vi "UDP_Packet_Inquiry.vi"(10 "Remote Port":u16=61557, 11 "UDP_Packet":T2 {"Command" format="%.0x"}) -> (2 "List":T1(array[cluster]) {"AmpUnit" format="%.0x"; "AnalogCH" format="%.0x"; "USB" format="%.0x"; "IP_Busy" format="%.0x"; "Count" format="%.0x"})   [LabVIEW 2017]
uses:
  UDP_Packet.ctl
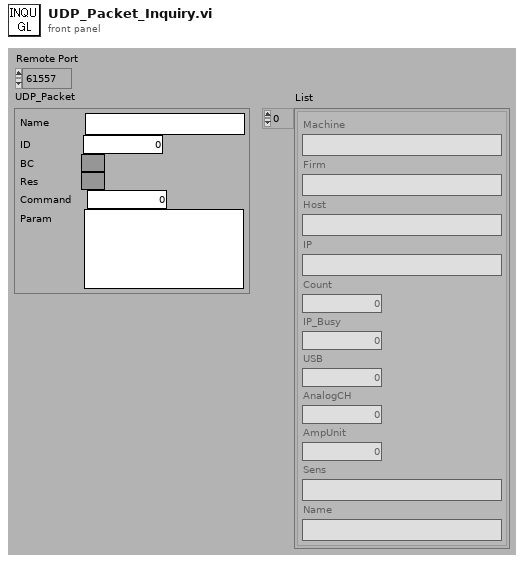
[diagram p1: front panel]
types:
  T1 = cluster{"Machine":string, "Firm":string, "Host":string, "IP":string, "Count":u32, "IP_Busy":u32, "USB":u32, "AnalogCH":u32, "AmpUnit":u32, "Sens":string, "Name":string}[]
  T2 = typedef "UDP_Packet.ctl" = cluster{"Name":string, "ID":u32, "BC":bool, "Res":bool, "Command":u32, "Param":string}
  T3 = enum16{"GL800", "GL200", "TH", "VT", "AC", "AT", "LU", "CO2", "TSR", "CO2_TH", "CO2_LU", "LU_TH"}[]
  T4 = cluster{"time":timestamp, "Inquiry":cluster{"Machine":string, "Firm":string, "Host":string, "IP":cluster{"A":u8, "B":u8, "C":u8, "D":u8}, "Count":u32, "IP_Busy":u32, "USB":u32, "AnalogCH":u32, "AmpUnit":u32, "Sens":cluster{"ID1":u16, "ID2":u16}, "Name":string}}
  T5 = cluster{"Machine":string, "Firm":string, "Host":string, "IP":cluster{"A":u8, "B":u8, "C":u8, "D":u8}, "Count":u32, "IP_Busy":u32, "USB":u32, "AnalogCH":u32, "AmpUnit":u32, "Sens":cluster{"ID1":u16, "ID2":u16}, "Name":string}
  T6 = cluster{timestamp, "Inquiry":cluster{"Machine":string, "Firm":string, "Host":string, "IP":cluster{"A":u8, "B":u8, "C":u8, "D":u8}, "Count":u32, "IP_Busy":u32, "USB":u32, "AnalogCH":u32, "AmpUnit":u32, "Sens":cluster{"ID1":u16, "ID2":u16}, "Name":string}}
  T7 = cluster{"time":timestamp, "Inquiry":cluster{"Machine":string, "Firm":string, "Host":string, "IP":cluster{"A":u8, "B":u8, "C":u8, "D":u8}, "Count":u32, "IP_Busy":u32, "USB":u32, "AnalogCH":u32, "AmpUnit":u32, "Sens":cluster{"ID1":u16, "ID2":u16}, "Name":string}}[]
  T8 = cluster{"Host":string, "IP":cluster{"A":u8, "B":u8, "C":u8, "D":u8}}
  T9 = cluster{"Machine":string, "Host":string, "IP":cluster{"A":u8, "B":u8, "C":u8, "D":u8}, "Inquiry":cluster{"Machine":string, "Firm":string, "Host":string, "IP":cluster{"A":u8, "B":u8, "C":u8, "D":u8}, "Count":u32, "IP_Busy":u32, "USB":u32, "AnalogCH":u32, "AmpUnit":u32, "Sens":cluster{"ID1":u16, "ID2":u16}, "Name":string}}
  T10 = cluster{"Machine":string, "Host":string, "IP":cluster{"A":u8, "B":u8, "C":u8, "D":u8}, "Inquiry":cluster{"Machine":string, "Firm":string, "Host":string, "IP":cluster{"A":u8, "B":u8, "C":u8, "D":u8}, "Count":u32, "IP_Busy":u32, "USB":u32, "AnalogCH":u32, "AmpUnit":u32, "Sens":cluster{"ID1":u16, "ID2":u16}, "Name":string}}[]
  T11 = cluster{"Machine":string, "Firm":string, "Host":string, string, "Count":u32, "IP_Busy":u32, "USB":u32, "AnalogCH":u32, "AmpUnit":u32, string, "Name":string}
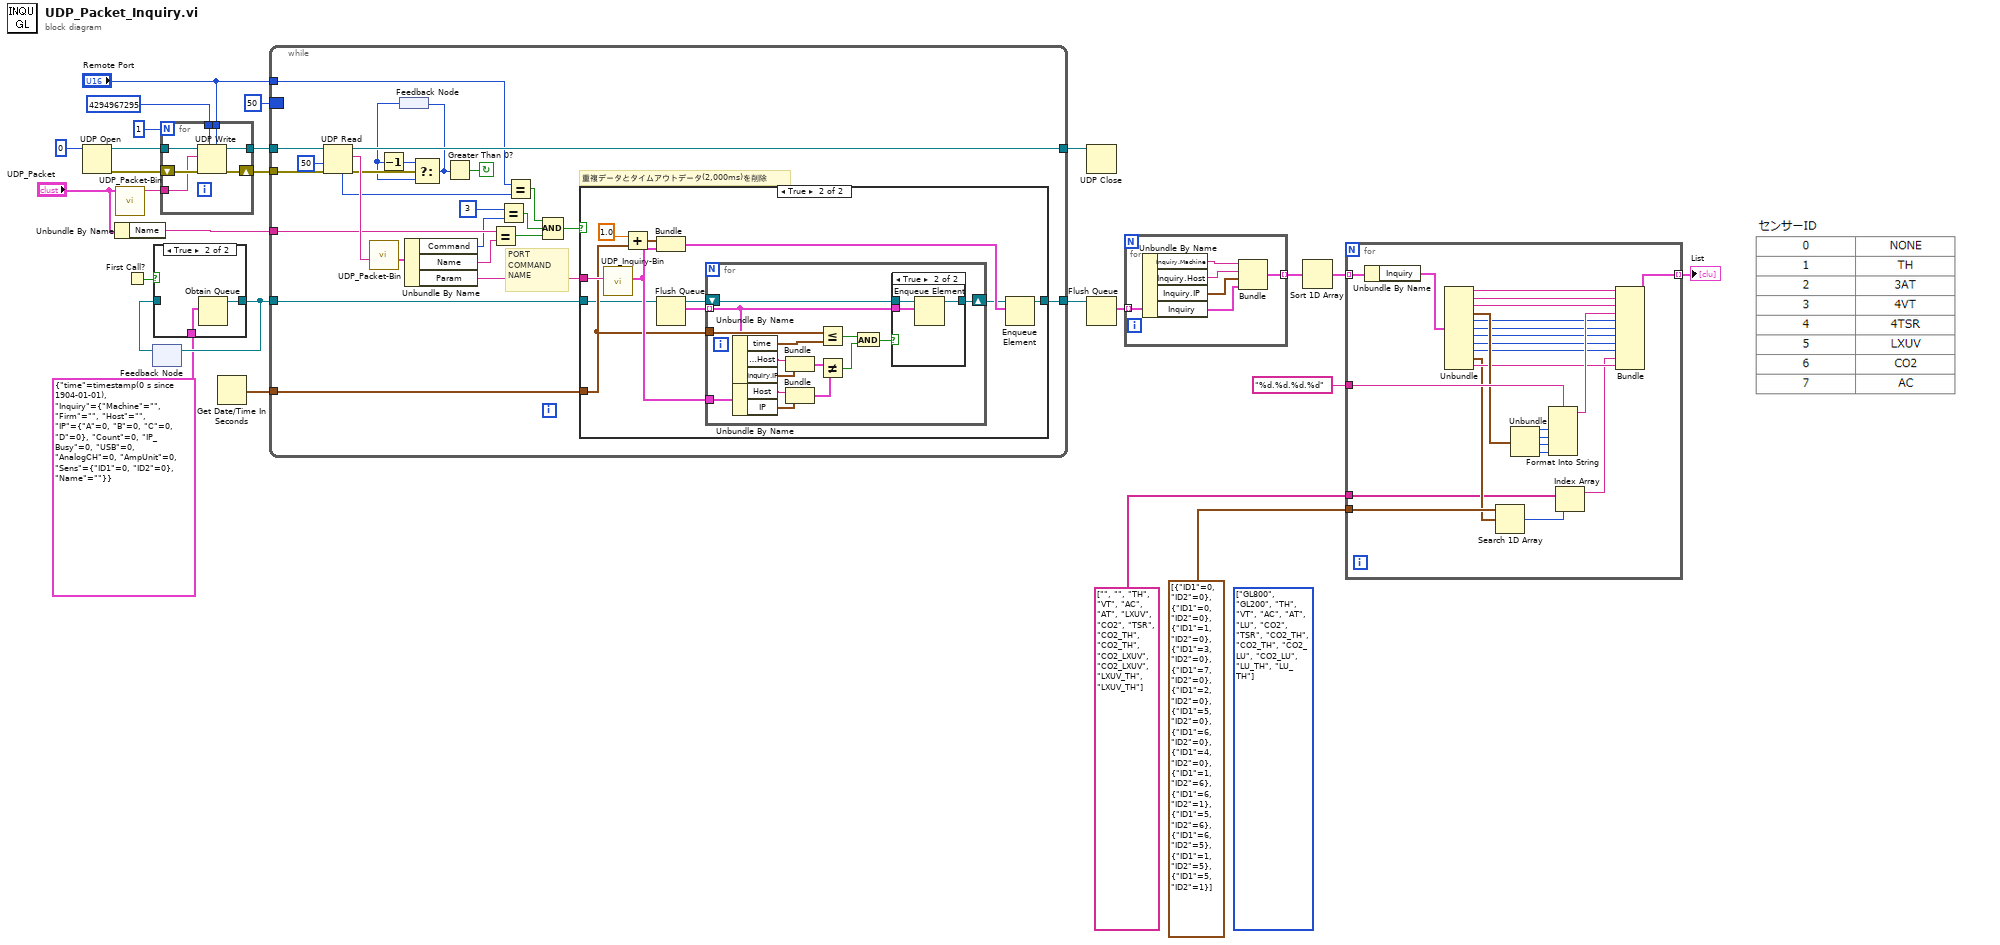
[diagram p0: block diagram]
diagram:
  (unwired) T3 [enum."GL800", enum."GL200", enum."TH", enum."VT", enum."AC", enum."AT", enum."LU", enum."CO2", enum."TSR", enum."CO2_TH", enum."CO2_TH", enum."CO2_LU", enum."CO2_LU", enum."LU_TH", enum."LU_TH"] items=["GL800", "GL200", "TH", "VT", "AC", "AT", "LU", "CO2", "TSR", "CO2_TH", "CO2_LU", "LU_TH"]
  n1 = UDP Open(11:u16 0 ("port")) -> (port=w26:refnum<k16>, 0:w25:errorcluster)  [unwired: 1 in, 4 out]
  n2 = Unbundle By Name("UDP_Packet") -> ("Name"=w16:string)
  n3 = call "UDP_Packet-Bin.vi"("IN_Packet"="UDP_Packet") -> ("OUT_BIN"=w22:string)  [unwired: 1 in, 9 out]
  n4 = First Call?() -> (First Call?: T/F=w14:bool)
  n5 = feedback #1() -> (w15:refnum<queue>)  [unwired: 1 out]
  n6 = case shown="TRUE" w14 {
    tunnel: [w27 w29] -> w12
    tunnel: w15 -> [w27 _]
    tunnel: T4 {"time"=timestamp(0 s since 1904-01-01), "Inquiry"={"Machine"="", "Firm"="", "Host"="", "IP"={"A"=0, "B"=0, "C"=0, "D"=0}, "Count"=0, "IP_Busy"=0, "USB"=0, "AnalogCH"=0, "AmpUnit"=0, "Sens"={"ID1"=0, "ID2"=0}, "Name"=""}} ("Inquiry") -> [_ w28]
    frame False {
    }
    frame True {
      n7 = Obtain Queue(element data type=w28) -> (queue out=w29:refnum<queue>)  [unwired: 3 in, 3 out]
    }
  }
  n8 = feedback-in #1(w12) -> ()
  n9 = for {
    N: 1 -> [_]
    tunnel: w26 -> [w34]
    tunnel: u32 4294967295 -> [w36]
    tunnel: "Remote Port" -> [w35]
    shift-right: [w32] -> w19
    shift-left: w25 -> [w33]
    tunnel: [w31] -> w20
    tunnel: w22 -> [w30]
    n10 = UDP Write(address=w36, port or service name=w35, connection ID=w34, data in=w30, 8:w33) -> (error out=w32:errorcluster, 3:w31:refnum<k16>)  [unwired: 1 out]
  }
  n11 = Get Date/Time In Seconds() -> (seconds since 1Jan1904=w10:timestamp)
  n12 = while {
    tunnel: [w61] -> w21
    tunnel: w20 -> [w60]
    tunnel: w19 -> [w59]
    tunnel: "Remote Port" -> [w52]
    tunnel: w16 -> [w50]
    tunnel: [w43] -> w13
    tunnel: w12 -> [w44]
    border: i16 50 -> [_]
    tunnel: w10 -> [w37]
    stop <- w38 continue-if-true
    # "重複データとタイムアウトデータ(2,000ms)を削除"
    # "PORT\nCOMMAND\nNAME"
    n13 = UDP Read(connection ID=w60, timeout ms (25000)=50, 8:w59) -> (data out=w57:string, error out=w42:errorcluster, 3:w61:refnum<k16>, 4:w53:u16)  [unwired: 2 out]
    n14 = call "UDP_Packet-Bin.vi"("IN_BIN"=w57) -> ("OUT_Packet"=w56:T2)  [unwired: 1 in, 9 out]
    n15 = feedback #2() -> (w41:i16)
    n16 = Decrement(x=w41) -> (x-1=w40:i16)
    n17 = Unbundle By Name(w56) -> ("Command"=w47:u32, "Name"=w49:string, "Param"=w45:string)
    n18 = Select(t=w40, s=w42, f=w41) -> (s? t:f=w39:i16)
    n19 = feedback-in #2(w39) -> ()
    n20 = Greater Than 0?(x=w39) -> (x > 0?=w38:bool)
    n21 = Equal?(x=w50, y=w49) -> (x = y?=w55:bool)
    n22 = Equal?(x=u32 3 ("y"), y=w47) -> (x = y?=w51:bool)
    n23 = Equal?(x=w52, y=w53) -> (x = y?=w54:bool)
    n24 = Compound Arithmetic op=AND(w54, w51, w55) -> (w46:bool)
    n25 = case shown="TRUE" w46 {
      tunnel: w45 -> [_ w73]
      tunnel: w44 -> [w62 w65]
      tunnel: [w62 w72] -> w43
      tunnel: w37 -> [_ w68]
      frame False {
      }
      frame True {
        n26 = call "UDP_Inquiry-Bin.vi"("IN_Param"=w73) -> ("Inquiry"=w71:T5)  [unwired: 10 out]
        n27 = Add(x=1.0, y=w68) -> (x+y=w67:timestamp)
        n28 = Bundle(w67, "Inquiry"=w71) -> (w70:T6)  [unwired: 1 out]
        n29 = Flush Queue(queue=w65) -> (queue out=w64:refnum<queue>, remaining elements=w63:T7)  [unwired: 1 in, 1 out]
        n30 = for {
          tunnel: w63 -> [w83] mode=indexing
          tunnel: w71 -> [w88]
          shift-right: [w85] -> w69
          shift-left: w64 -> [w84]
          tunnel: w68 -> [w86]
          n31 = Unbundle By Name(w83) -> ("time"=w87:timestamp, "Inquiry.Host"=w78:string, "Inquiry.IP"=w79:cluster{"A":u8, "B":u8, "C":u8, "D":u8})
          n32 = Unbundle By Name(w88) -> ("Host"=w76:string, "IP"=w75:cluster{"A":u8, "B":u8, "C":u8, "D":u8})
          n33 = Bundle("Host"=w78, "IP"=w79) -> (w77:T8)  [unwired: 1 out]
          n34 = Bundle("Host"=w76, "IP"=w75) -> (w74:T8)  [unwired: 1 out]
          n35 = Less Or Equal?(x=w86, y=w87) -> (x <= y?=w81:bool)
          n36 = Not Equal?(x=w77, y=w74) -> (x != y?=w82:bool)
          n37 = And(x=w81, y=w82) -> (x .and. y?=w80:bool)
          n38 = case shown="TRUE" w80 {
            tunnel: [w89 w91] -> w85
            tunnel: w84 -> [w89 w92]
            tunnel: w83 -> [_ w90]
            frame False {
            }
            frame True {
              n39 = Enqueue Element(queue=w92, element=w90) -> (queue out=w91:refnum<queue>)  [unwired: 1 in, 3 out]
            }
          }
        }
        n40 = Enqueue Element(queue=w69, element=w70) -> (queue out=w72:refnum<queue>)  [unwired: 1 in, 3 out]
      }
    }
  }
  n41 = UDP Close(connection ID=w21) -> ()  [unwired: 1 in, 2 out]
  n42 = Flush Queue(queue=w13) -> (remaining elements=w8:T7)  [unwired: 1 in, 2 out]
  n43 = for {
    tunnel: w8 -> [w98] mode=indexing
    tunnel: [w94] -> w7 mode=indexing
    n44 = Unbundle By Name(w98) -> ("Inquiry.Machine"=w93:string, "Inquiry.Host"=w96:string, "Inquiry.IP"=w95:cluster{"A":u8, "B":u8, "C":u8, "D":u8}, "Inquiry"=w97:T5)
    n45 = Bundle("Machine"=w93, "Host"=w96, "IP"=w95, "Inquiry"=w97) -> (w94:T9)  [unwired: 1 out]
  }
  n46 = Sort 1D Array(array=w7) -> (sorted array=w6:T10)
  n47 = for {
    tunnel: w6 -> [w122] mode=indexing
    tunnel: [w115] -> w5 mode=indexing
    tunnel: "%d.%d.%d.%d" ("format string") -> [w121]
    tunnel: cluster{"ID1":u16, "ID2":u16}[] [{"ID1"=0, "ID2"=0}, {"ID1"=0, "ID2"=0}, {"ID1"=1, "ID2"=0}, {"ID1"=3, "ID2"=0}, {"ID1"=7, "ID2"=0}, {"ID1"=2, "ID2"=0}, {"ID1"=5, "ID2"=0}, {"ID1"=6, "ID2"=0}, {"ID1"=4, "ID2"=0}, {"ID1"=1, "ID2"=6}, {"ID1"=6, "ID2"=1}, {"ID1"=5, "ID2"=6}, {"ID1"=6, "ID2"=5}, {"ID1"=1, "ID2"=5}, {"ID1"=5, "ID2"=1}] -> [w103]
    tunnel: string[] ["", "", "TH", "VT", "AC", "AT", "LXUV", "CO2", "TSR", "CO2_TH", "CO2_TH", "CO2_LXUV", "CO2_LXUV", "LXUV_TH", "LXUV_TH"] -> [w99]
    n48 = Unbundle By Name(w122) -> ("Inquiry"=w114:T5)
    n49 = Unbundle(w114) -> ("Machine"=w113:string, "Firm"=w112:string, "Host"=w111:string, "IP"=w110:cluster{"A":u8, "B":u8, "C":u8, "D":u8}, "Count"=w109:u32, "IP_Busy"=w108:u32, "USB"=w107:u32, "AnalogCH"=w106:u32, "AmpUnit"=w105:u32, "Sens"=w102:cluster{"ID1":u16, "ID2":u16}, "Name"=w104:string)
    n50 = Search 1D Array(1D array=w103, element=w102) -> (index of element=w100:i32)  [unwired: 1 in]
    n51 = Unbundle(w110) -> ("A"=w120:u8, "B"=w119:u8, "C"=w118:u8, "D"=w117:u8)
    n52 = Format Into String(format string=w121, w120, w119, w118, w117) -> (resulting string=w116:string)  [unwired: 2 in, 1 out]
    n53 = Index Array(array=w99, index=w100) -> (element=w101:string)
    n54 = Bundle("Machine"=w113, "Firm"=w112, "Host"=w111, w116, "Count"=w109, "IP_Busy"=w108, "USB"=w107, "AnalogCH"=w106, "AmpUnit"=w105, w101, "Name"=w104) -> (w115:T11)  [unwired: 1 out]
  }
  "List" <- w5
